vi "Read Digital Inptus.vi"(8 "error in":errorcluster, 11 "VISA Refnum in":refnum<visa-resource-name>) -> (0 "error out":errorcluster, 2 "Digital Inputs":bool[](array[boolean]), 3 "VISA Refnum out":refnum<visa-resource-name>)   [LabVIEW 2024, in "CTIWrapper.lvlib"]
uses:
  CTIWrapper.lvlib
  <instrlib>/HandsOnPi2040/Public/DigIns.ctl
  <instrlib>/HandsOnPi2040/HandsOnPi2040.lvlib
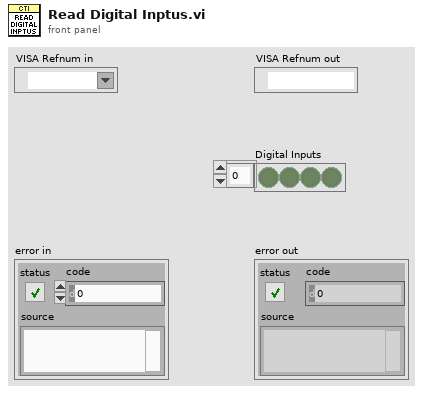
[diagram p1: front panel]
types:
  T1 = typedef "HandsOnPi2040.lvlib/DigIns.ctl" = enum16{"No DI - Error", "DI1 (GPIO7)", "DI2 (GPIO8)", "DI3 (GPIO9)", "DI4 (GPIO10)"}
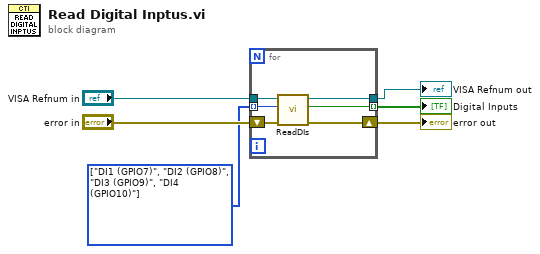
[diagram p0: block diagram]
diagram:
  w2 = T1[] [enum."DI1 (GPIO7)", enum."DI2 (GPIO8)", enum."DI3 (GPIO9)", enum."DI4 (GPIO10)"] items=["No DI - Error", "DI1 (GPIO7)", "DI2 (GPIO8)", "DI3 (GPIO9)", "DI4 (GPIO10)"] ("Array")
  n1 = for {
    tunnel: "VISA Refnum in" -> [w10]
    tunnel: [w9] -> w4
    tunnel: w2 -> [w8] mode=indexing
    tunnel: [w7] -> w1 mode=indexing
    shift-right: [w12] -> w5
    shift-left: "error in" -> [w11]
    n2 = call <instrlib>:"ReadDIs.vi"("error in (no error)"=w11, "Digital Inputs"=w8, "VISA resource name"=w10) -> ("error out"=w12:errorcluster, "DIStatus"=w7:bool, "VISA resource name out"=w9:refnum<visa-resource-name>)  [unwired: 6 in]
  }
  "VISA Refnum out" <- w4
  "Digital Inputs" <- w1
  "error out" <- w5
